vi "LVClass_HasoEngine AlignementDataFromImage.vi"(0 "HasoEngine in":refnum<class "HasoEngine.lvclass">, 5 "Image in":refnum<class "Image.lvclass">, 11 "error in (no error)":errorcluster) -> (4 "HasoEngine out":refnum<class "HasoEngine.lvclass">, 6 "barycentre":T1, 15 "error out":errorcluster)   [LabVIEW 2020, in "HasoEngine.lvclass"]
doc: "HasoSlopes computation preferences getter.\n\n--------------------------------------------------------------------------------\n\n<B>HasoEngineIn </B> : HasoEngine object.\n<B>HasoEngineOut </B> : HasoEngine object.\n<B>image </B> : Image object.\n<B>barycentre </B> : Barycenter coordinates.\n<B>ErrorIn </B> : Error\n<B>ErrorOut </B> : Error\n\n--------------------------------------------------------------------------------"
uses:
  HasoEngine.lvclass
  Image/Image.lvclass
  Controls/Point2Df.ctl
  HasoEngine.lvclass/HasoEngine.ctl
  Image/LVClass_Image read Image Compat ptr.vi
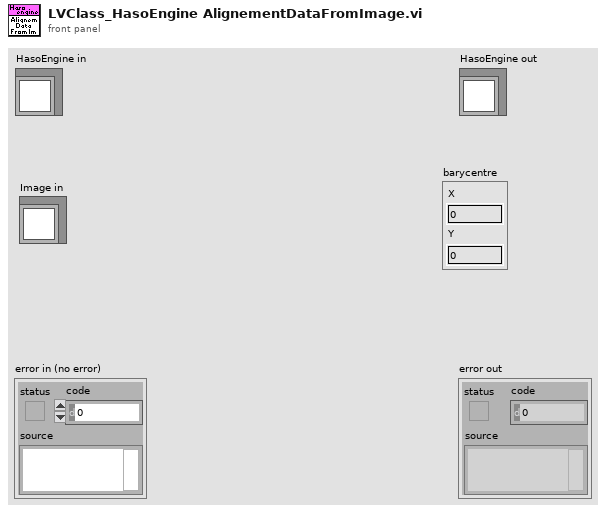
[diagram p1: front panel]
types:
  T1 = typedef "Point2Df.ctl" = cluster{"X":sgl, "Y":sgl}
  T2 = typedef "ClassID.ctl" = i64
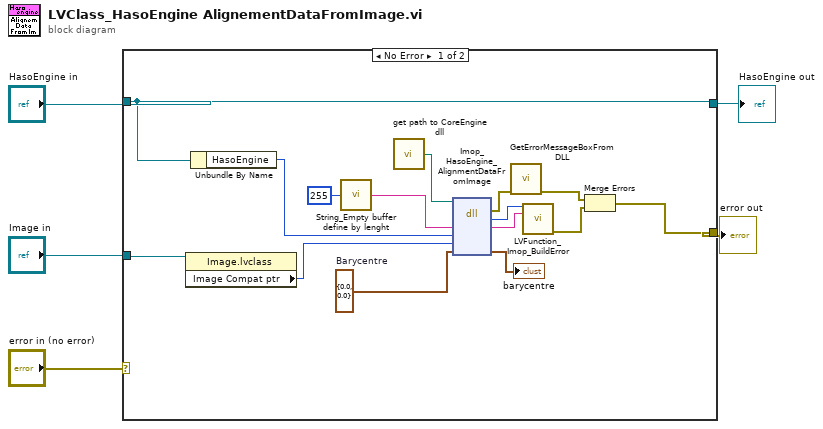
[diagram p0: block diagram]
diagram:
  n1 = case shown="No Error" "error in (no error)" {
    selector: "error in (no error)" -> [_ w21]
    tunnel: "HasoEngine in" -> [w13 w22]
    tunnel: [w13 w22] -> w2
    tunnel: [w6 w21] -> w3
    tunnel: "Image in" -> [w15 _]
    frame No Error {
      w11 = T1 {"X"=0.0, "Y"=0.0}  # Barycentre
      n2 = property class="Image.lvclass"(reference=w15) -> ("Image Compat ptr"=w14:T2)  [unwired: 1 in, 2 out]
      n3 = Unbundle By Name(w13) -> ("HasoEngine"=w12:T2)
      n4 = call "String_Empty buffer define by lenght.vi"("Lenght (255)"=255) -> ("Empty buffer"=w18:string)
      n5 = call "get path to CoreEngine dll.vi"() -> ("path to wavekit library"=w17:path)  [unwired: 14 in, 1 out]
      n6 = dll-call lib="D:/2_trunk/Soft_haso/ImOpCoreEngine4_LV2011/DLLs/ImopEngine4_vc100.dll" fn="Imop_HasoEngine_AlignmentDataFromImage"(path in=w17, "message"=w18, "objet"=w12, "Image"=w14, "barycentre"=w11) -> (error out=w16:errorcluster, "return type"=w19:i32, "message"=w20:string, "barycentre"=→"barycentre":T1)  [unwired: 4 in, 1 out]
      n7 = call "GetErrorMessageBoxFromDLL.vi"("error IN"=w16) -> ("error OUT"=w8:errorcluster)  [unwired: 10 in]
      n8 = call "LVFunction_Imop_BuildError.vi"("code"=w19, "String to Prepend to source (\"\")"=w20) -> ("error out"=w7:errorcluster)  [unwired: 13 in]
      n9 = Merge Errors(w8, w7) -> (w6:errorcluster)
    }
    frame Error {
    }
  }
  "error out" <- w3
  "HasoEngine out" <- w2
